vi "VI.get_control_lua.vi"(5 "LuaVIEW reference":T1) -> (15 "error out":errorcluster)   [LabVIEW 2012]
doc: "Gets the value of a control or indicator. Any data type that can be passed as compound data or occur as an element of compound data is supported.\nParameters:\nobj:self, VI object.\nstr:label, label of control/indicator whose value to get.\nResults:\nany:value, value of control/indicator.\nErrors:\nNot a VI object.\nDead VI object.\nNo such control or indicator.\nData type of control/indicator not supported."
uses:
  typedefs/t_LuaVIEW Reference.ctl
  subvis/private/LuaVIEW Pull (object).vi
  subvis/private/LuaVIEW Pull (string).vi
  subvis/private/LuaVIEW Push (flat data).vi
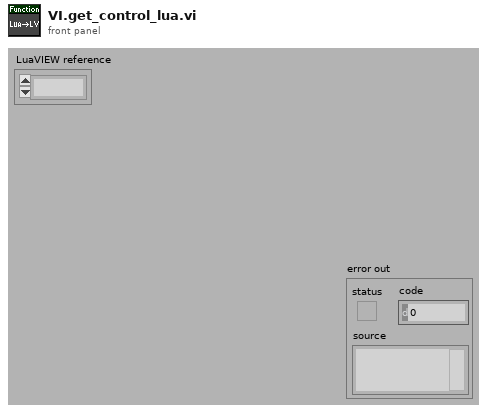
[diagram p1: front panel]
types:
  T1 = typedef "t_LuaVIEW Reference.ctl" = refnum<k1>
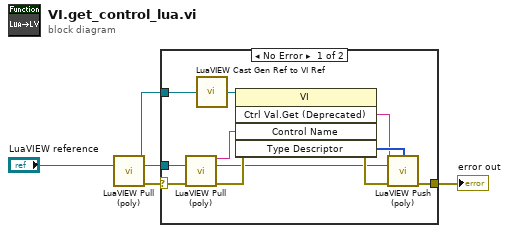
[diagram p0: block diagram]
diagram:
  n1 = call-poly "LuaVIEW Pull (poly).vi"("LuaVIEW reference in"="LuaVIEW reference") -> ("object refnum"=w3:refnum<vi>, "LuaVIEW reference out"=w1:T1, "error out"=w2:errorcluster)  [unwired: 11 in, 1 out]
  n2 = case shown="No Error" w2 {
    selector: w2 -> [w15 w17]
    tunnel: [w6 w17] -> w4
    tunnel: w3 -> [w16 _]
    tunnel: w1 -> [w14 _]
    frame No Error {
      n3 = call-poly "LuaVIEW Pull (poly).vi"("LuaVIEW reference in"=w14, "error in (no error)"=w15) -> ("string"=w8:string, "LuaVIEW reference out"=w9:T1, "error out"=w12:errorcluster)  [unwired: 11 in]
      n4 = call "LuaVIEW Cast Gen Ref to VI Ref.vi"("refnum in"=w16) -> ("refnum out"=w13:refnum<vi>)  [unwired: 14 in]
      n5 = invoke class="VI" method="Ctrl Val.Get (Deprecated)"(reference=w13, error in=w12, "Control Name"=w8) -> (error out=w11:errorcluster, "Get Control Value"=w7:string, "Type Descriptor"=w10:i16[])  [unwired: 2 in, 2 out]
      n6 = call-poly "LuaVIEW Push (poly).vi"("flat data"=w7, "type descriptor"=w10, "LuaVIEW reference in"=w9, "error in (no error)"=w11) -> ("error out"=w6:errorcluster)  [unwired: 10 in, 1 out]
    }
    frame Error {
    }
  }
  "error out" <- w4
